vi "Config.Merge SW Items.vi"(9 "SW Items":string[][](array[string]), 11 "SW List In":string[][](array[string])) -> (1 "Modified":bool, 3 "SW List Out":string[][](array[string]))   [LabVIEW 2024, in "EQMF.lvlib" / "Config Utils.lvlib"]
doc: "This VI inputs two 2D arrays of string that are the SW item lists and merges the two. Any item from SW List In that matches with SW Items is over written by the SW Items record.\n\nINPUTS:\n<B>SW Items In</B> - The existing SW Item List.\n<B>SW Items</B> - New SW Item List\n\nOUTPUTS:\n<B>Modified</B> - TRUE indicates that one or more name was already in the SW item list and those records have been updated.\n\nERRORS: \nN/A"
uses:
  Config Utils.lvlib
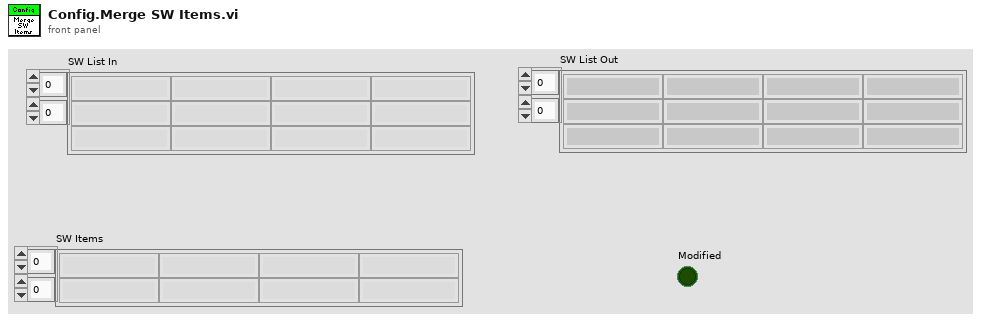
[diagram p1: front panel]
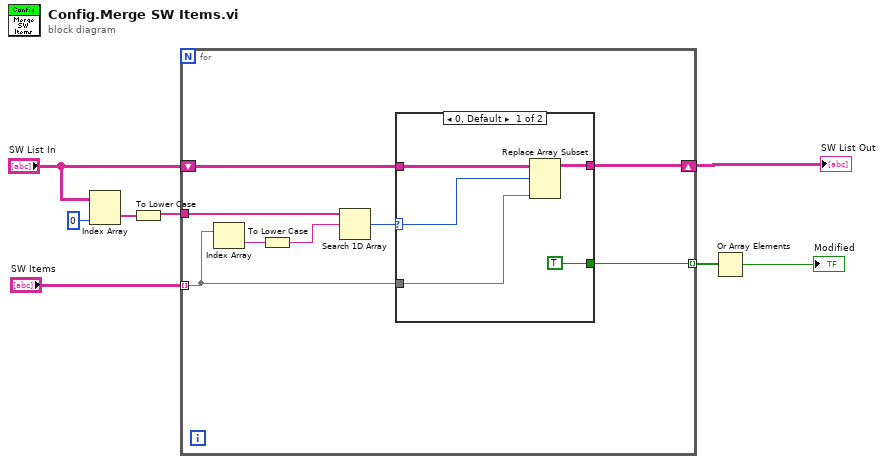
[diagram p0: block diagram]
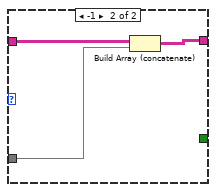
[diagram p2: hidden frame]
diagram:
  n1 = Index Array(array="SW List In", index (col)=0 ("index")) -> (element=w7:string[])  [unwired: 1 in]
  n2 = To Lower Case(string=w7) -> (all lower case string=w6:string[])
  n3 = for {
    tunnel: w6 -> [w12]
    shift-right: [w13] -> w4
    shift-left: "SW List In" -> [w14]
    tunnel: "SW Items" -> [w10] mode=indexing
    tunnel: [w9] -> w2 mode=indexing
    n4 = Index Array(array=w10) -> (element=w11:string)  [unwired: 1 in]
    n5 = To Lower Case(string=w11) -> (all lower case string=w16:string)
    n6 = Search 1D Array(1D array=w12, element=w16) -> (index of element=w15:i32)  [unwired: 1 in]
    n7 = case shown="0, Default" w15 {
      selector: w15 -> [w19 _]
      tunnel: w14 -> [w21 w24]
      tunnel: [w20 w23] -> w13
      tunnel: w10 -> [w18 w22]
      tunnel: [TRUE _] -> w9
      frame 0, Default {
        n8 = Replace Array Subset(array=w21, new element=w18, index (row)=w19) -> (w20:string[][])  [unwired: 1 in]
      }
      frame -1 {
        n9 = Build Array (concatenate)(w24, w22) -> (w23:string[][])
      }
    }
  }
  "SW List Out" <- w4
  n10 = Or Array Elements(Boolean array=w2) -> (logical OR=→"Modified":bool)
